vi "Get Columns from Query.vi"(8 "error in (no error)":errorcluster, 11 "Query":string) -> (0 "error out":errorcluster, 2 "COLHEADERS":string[](array[string]), 3 "Array":string[](array[string]))   [LabVIEW 2020]
uses:
  <vilib>/Utility/error.llb/whitespace.ctl
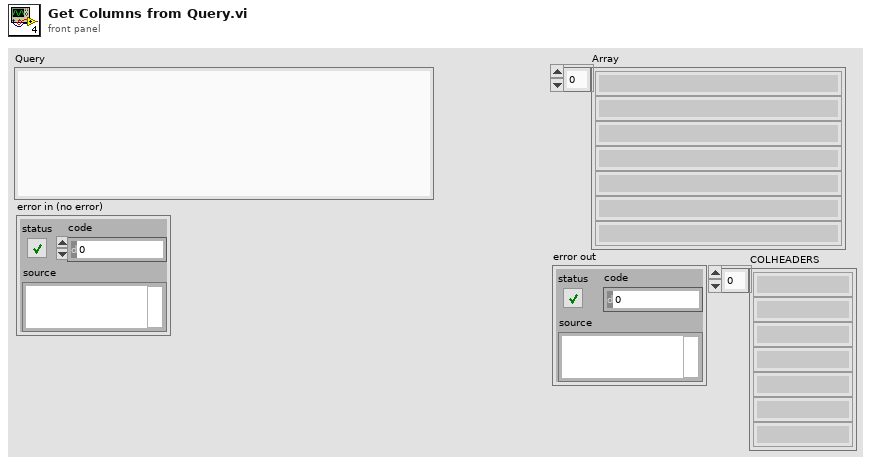
[diagram p1: front panel]
types:
  T1 = typedef "whitespace.ctl" = u16
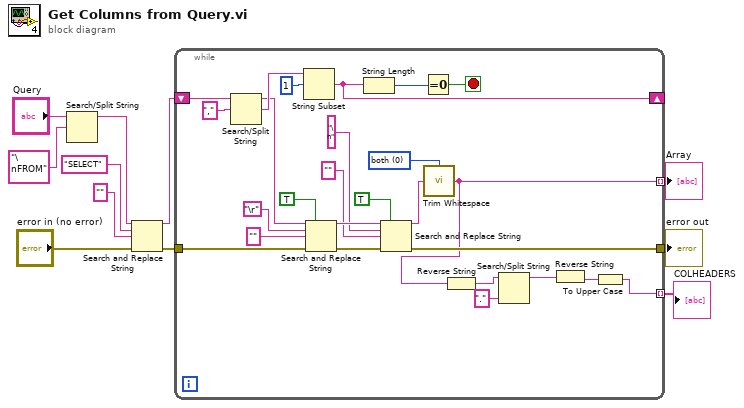
[diagram p0: block diagram]
diagram:
  n1 = Search/Split String(string="Query", search string/char (-)="\nFROM") -> (substring before match=w10:string)  [unwired: 1 in, 2 out]
  n2 = Search and Replace String(input string=w10, search string="SELECT", replace string="" ("replace string (\"\")"), error in="error in (no error)") -> (result string=w7:string, error out=w3:errorcluster)  [unwired: 4 in, 2 out]
  n3 = while {
    tunnel: [w14] -> w6 mode=indexing
    shift-right: [w31] -> _
    shift-left: w7 -> [w37]
    tunnel: [w21] -> w4
    tunnel: w3 -> [w20]
    tunnel: [w12] -> w1 mode=indexing
    stop <- w32 stop-if-true
    w22 = T1 0 items=["both", "start of string", "end of string"] ("location (both)")
    n4 = Search/Split String(string=w37, search string/char (-)=",") -> (substring before match=w30:string, match + rest of string=w35:string)  [unwired: 1 in, 1 out]
    n5 = String Subset(string=w35, offset (0)=1) -> (substring=w31:string)  [unwired: 1 in]
    n6 = Search and Replace String(replace all?=TRUE ("replace all? (F)"), input string=w30, search string="\r", replace string="" ("replace string (\"\")"), error in=w20) -> (result string=w26:string, error out=w18:errorcluster)  [unwired: 3 in, 2 out]
    n7 = String Length(string=w31) -> (length=w33:i32)
    n8 = Search and Replace String(replace all?=TRUE ("replace all? (F)"), input string=w26, search string="\n", replace string="" ("replace string (\"\")"), error in=w18) -> (result string=w23:string, error out=w21:errorcluster)  [unwired: 3 in, 2 out]
    n9 = Equal To 0?(x=w33) -> (x = 0?=w32:bool)
    n10 = call <vilib>:"Trim Whitespace.vi"("string"=w23, "location (both)"=w22) -> ("trimmed string"=w14:string)
    n11 = Reverse String(1:w14) -> (0:w17:string)
    n12 = Search/Split String(string=w17, search string/char (-)=".") -> (substring before match=w15:string)  [unwired: 1 in, 2 out]
    n13 = Reverse String(1:w15) -> (0:w13:string)
    n14 = To Upper Case(1:w13) -> (0:w12:string)
  }
  "Array" <- w6
  "error out" <- w4
  "COLHEADERS" <- w1
